vi "determine Warnings (subVI).vi"(8 "error in (no error)":errorcluster, 9 "Min Temp":dbl, 10 "Max Temp":dbl, 11 "Current Temp":dbl) -> (0 "error out":errorcluster, 1 "Warning?":bool, 2 "Warning Text":string="Freeze Warning")   [LabVIEW 2014]
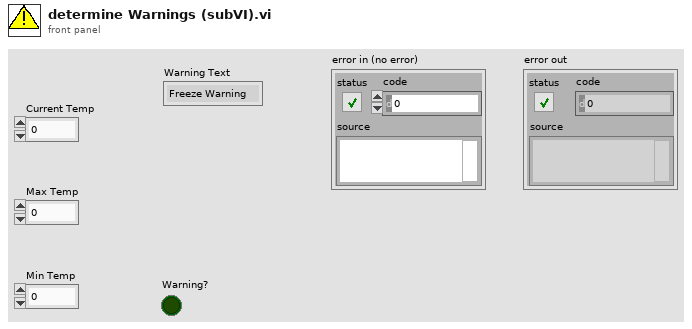
[diagram p1: front panel]
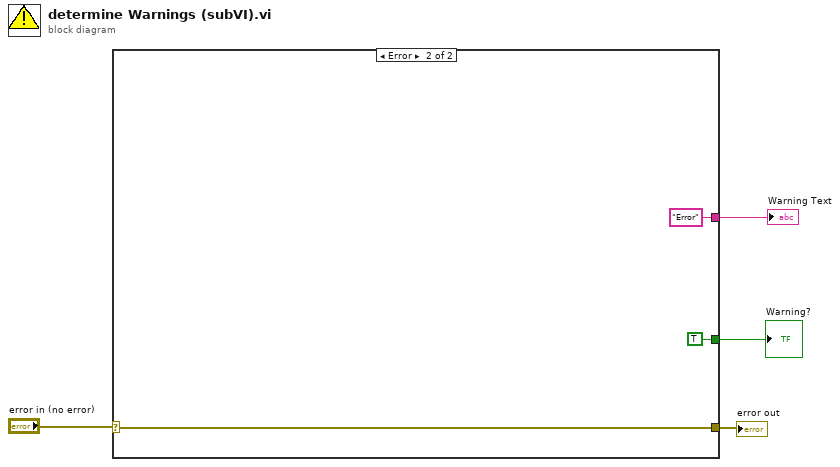
[diagram p0: block diagram]
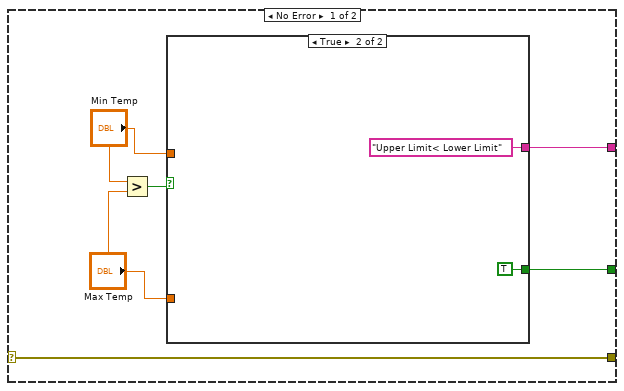
[diagram p2: hidden frame]
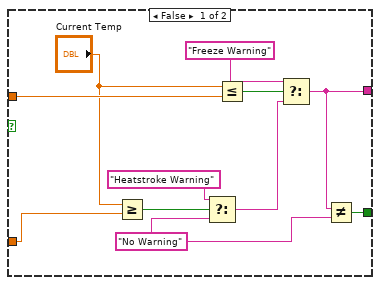
[diagram p3: hidden frame]
diagram:
  n1 = case shown="Error" "error in (no error)" {
    selector: "error in (no error)" -> [w5 w26]
    tunnel: [w10 "Error" ("Warning Text")] -> w4
    tunnel: [w9 TRUE] -> w3
    tunnel: [w5 w26] -> w1
    frame No Error {
      n2 = Greater?(x="Min Temp", y="Max Temp") -> (0:w8:bool)
      n3 = case shown="True" w8 {
        tunnel: [w15 "Upper Limit< Lower Limit" ("Warning Text")] -> w10
        tunnel: [w14 TRUE] -> w9
        tunnel: "Max Temp" -> [w13 _]
        tunnel: "Min Temp" -> [w12 _]
        frame False {
          w16 = "No Warning" ("Warning Text")
          n4 = Greater Or Equal?(x="Current Temp", y=w13) -> (x >= y?=w21:bool)
          n5 = Select(t="Heatstroke Warning" ("Warning Text"), s=w21, f=w16) -> (s? t:f=w17:string)
          n6 = Less Or Equal?(x="Current Temp", y=w12) -> (x <= y?=w19:bool)
          n7 = Select(t="Freeze Warning" ("Warning Text"), s=w19, f=w17) -> (s? t:f=w15:string)
          n8 = Not Equal?(x=w15, y=w16) -> (x != y?=w14:bool)
        }
        frame True {
        }
      }
    }
    frame Error {
    }
  }
  "Warning?" <- w3
  "Warning Text" <- w4
  "error out" <- w1
